vi "Assigned instruments to class.vi"(8 "error in (no error)":errorcluster, 11 "Test Framework in":refnum<class "Test Framework.lvclass">) -> (0 "error out":errorcluster, 3 "Test Framework out":refnum<class "Test Framework.lvclass">)   [LabVIEW 2020, in "Test Framework.lvclass"]
uses:
  Test Framework.lvclass
  Instruments/Instrument.lvclass
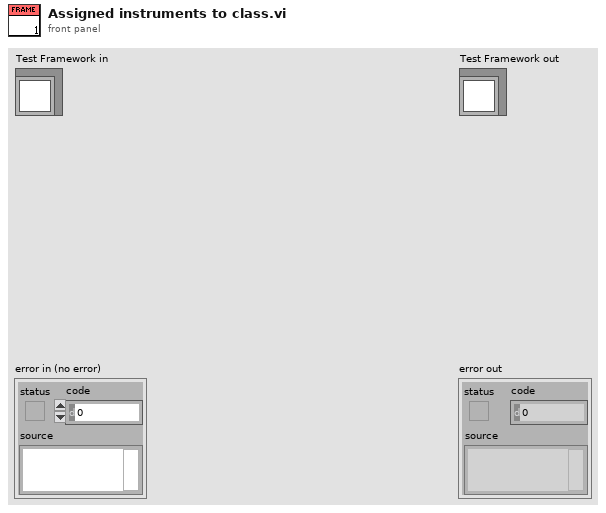
[diagram p1: front panel]
types:
  T1 = cluster{"Instrument Name":string, "Instrument.lvclass":refnum<class "Instrument.lvclass">}
  T2 = typedef "Test Framework.lvclass/Reference Selector.ctl" = enum16{"Signal Generator 1", "Signal Generator 2", "Spectrum Analyzer"}
  T3 = cluster{"Found Instruments":string[][], "Reference Selected":T2}
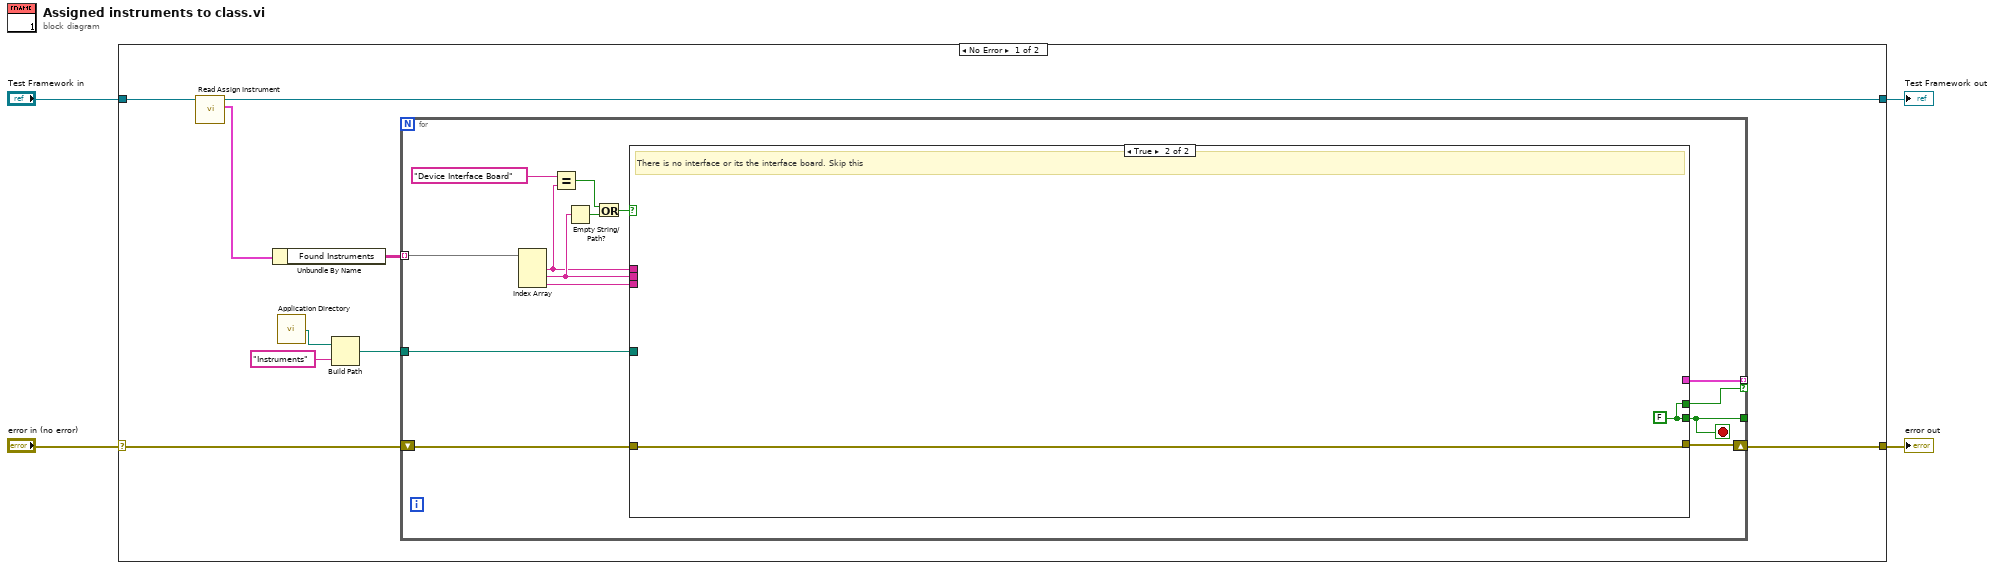
[diagram p0: block diagram]
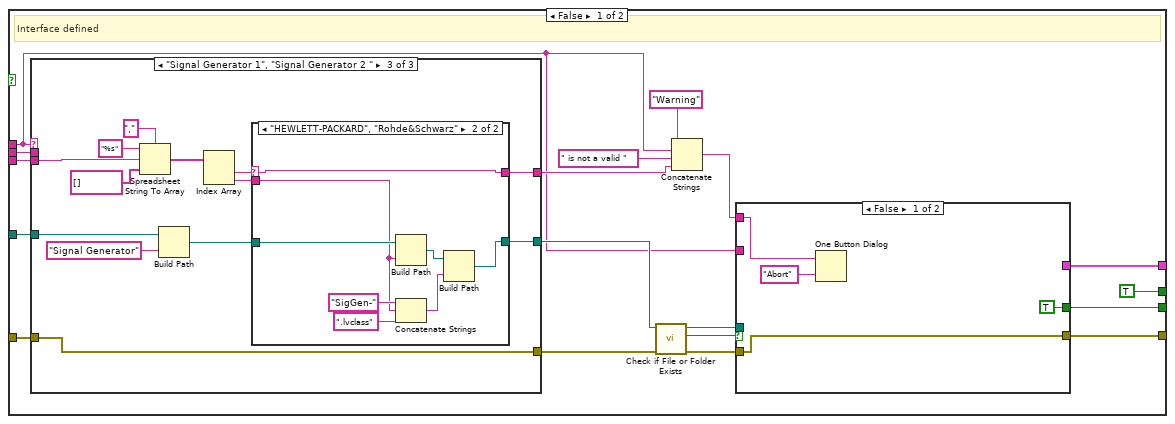
[diagram p2: hidden frame]
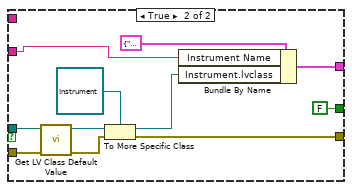
[diagram p3: hidden frame]
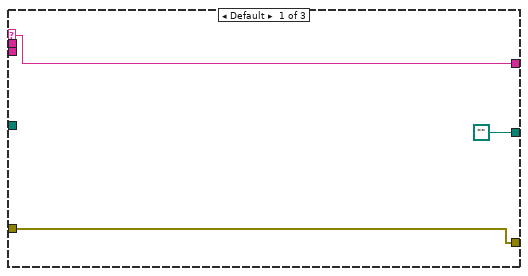
[diagram p4: hidden frame]
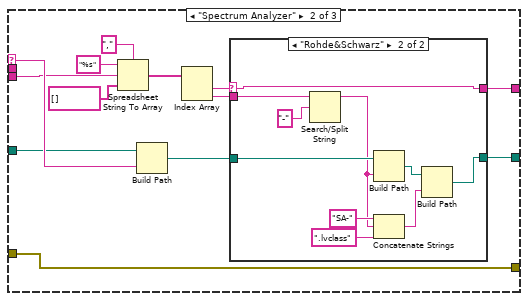
[diagram p5: hidden frame]
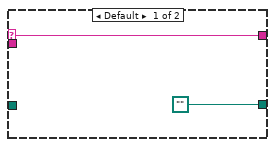
[diagram p6: hidden frame]
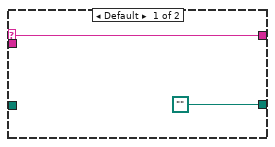
[diagram p7: hidden frame]
diagram:
  n1 = case shown="No Error" "error in (no error)" {
    selector: "error in (no error)" -> [w11 w115]
    tunnel: [w5 w115] -> w3
    tunnel: [w7 w114] -> w1
    tunnel: "Test Framework in" -> [w13 w114]
    frame No Error {
      n2 = call-dynamic "Read Assign Instrument.vi"("Test Framework in"=w13) -> ("Assign Instrument"=w6:T3, "Test Framework out"=w7:refnum<class "Test Framework.lvclass">)  [unwired: 9 in]
      n3 = Unbundle By Name(w6) -> ("Found Instruments"=w12:string[][])
      n4 = call <vilib>:"Application Directory.vi"() -> ("Application Directory"=w10:path)
      n5 = Build Path(base path=w10, name or relative path="Instruments") -> (appended path=w8:path)
      n6 = for {
        tunnel: w12 -> [w27] mode=indexing
        shift-right: [w21] -> w5
        shift-left: w11 -> [w25]
        tunnel: w8 -> [w24]
        tunnel: [w19] -> _
        tunnel: [w20] -> _ mode=indexing if=w18
        stop <- w19 stop-if-true
        n7 = Index Array(array=w27) -> (element #1=w17:string, element #2=w22:string, element #3=w26:string)  [unwired: 3 in]
        n8 = Equal?(x="Device Interface Board", y=w17) -> (x = y?=w14:bool)
        n9 = Empty String/Path?(string/path=w22) -> (empty?=w23:bool)
        n10 = Or(x=w14, y=w23) -> (x .or. y?=w15:bool)
        n11 = case shown="True" w15 {
          tunnel: w17 -> [w30 _]
          tunnel: w22 -> [w45 _]
          tunnel: w26 -> [w44 _]
          tunnel: w25 -> [w43 w113]
          tunnel: w24 -> [w42 _]
          tunnel: [w36 w113] -> w21
          tunnel: [w31 w112] -> w19
          tunnel: [w29 _] -> w20
          tunnel: [TRUE w112] -> w18
          frame False {
            # "Interface defined"
            n12 = case shown="\"Signal Generator 1\", \"Signal Generator 2 \"" w30 {
              selector: w30 -> [w63 w76 _]
              tunnel: w45 -> [_ _ _]
              tunnel: w44 -> [_ w74 w100]
              tunnel: w43 -> [w61 w65 w91]
              tunnel: w42 -> [_ w75 w101]
              tunnel: [path "" w66 w92] -> w40
              tunnel: [w61 w65 w91] -> w41
              tunnel: [w63 w64 w90] -> w33
              frame Default {
              }
              frame "Spectrum Analyzer" {
                n13 = Spreadsheet String To Array(delimiter (Tab)=",", format string="%s", spreadsheet string=w74, array type (2D Dbl)=string[] []) -> (array=w70:string[])
                n14 = Build Path(base path=w75, name or relative path=w76) -> (appended path=w67:path)
                n15 = Index Array(array=w70) -> (element #1=w69:string, element #2=w68:string)  [unwired: 2 in]
                n16 = case shown="\"Rohde&Schwarz\"" w69 {
                  selector: w69 -> [w77 w79]
                  tunnel: w68 -> [_ w88]
                  tunnel: w67 -> [_ w86]
                  tunnel: [path "" w80] -> w66
                  tunnel: [w77 w79] -> w64
                  frame Default {
                  }
                  frame "Rohde&Schwarz" {
                    n17 = Search/Split String(string=w88, search string/char (-)="-") -> (substring before match=w82:string)  [unwired: 1 in, 2 out]
                    n18 = Build Path(base path=w86, name or relative path=w82) -> (appended path=w85:path)
                    n19 = Concatenate Strings("SA-" ("string"), w82, ".lvclass" ("string")) -> (w84:string)
                    n20 = Build Path(base path=w85, name or relative path=w84) -> (appended path=w80:path)
                  }
                }
              }
              frame "Signal Generator 1", "Signal Generator 2 " {
                n21 = Spreadsheet String To Array(delimiter (Tab)=",", format string="%s", spreadsheet string=w100, array type (2D Dbl)=string[] []) -> (array=w96:string[])
                n22 = Build Path(base path=w101, name or relative path="Signal Generator") -> (appended path=w93:path)
                n23 = Index Array(array=w96) -> (element #1=w95:string, element #2=w94:string)  [unwired: 2 in]
                n24 = case shown="\"HEWLETT-PACKARD\", \"Rohde&Schwarz\"" w95 {
                  selector: w95 -> [w102 w105]
                  tunnel: w94 -> [_ w104]
                  tunnel: w93 -> [_ w111]
                  tunnel: [path "" w106] -> w92
                  tunnel: [w102 w105] -> w90
                  frame Default {
                  }
                  frame "HEWLETT-PACKARD", "Rohde&Schwarz" {
                    n25 = Build Path(base path=w111, name or relative path=w104) -> (appended path=w110:path)
                    n26 = Concatenate Strings("SigGen-" ("string"), w104, ".lvclass" ("string")) -> (w109:string)
                    n27 = Build Path(base path=w110, name or relative path=w109) -> (appended path=w106:path)
                  }
                }
              }
            }
            n28 = call <vilib>:"Check if File or Folder Exists.vi"("error in (no error)"=w41, "path"=w40) -> ("error out"=w37:errorcluster, "file or folder exists?"=w39:bool, "dup path"=w38:path)  [unwired: 7 in]
            n29 = Concatenate Strings("Warning" ("string"), w30, " is not a valid " ("string"), w33) -> (w32:string)
            n30 = case shown="False" w39 {
              tunnel: w38 -> [_ w60]
              tunnel: w37 -> [w49 w59]
              tunnel: [w49 w55] -> w36
              tunnel: w32 -> [w48 _]
              tunnel: [TRUE FALSE] -> w31
              tunnel: w30 -> [_ w52]
              tunnel: [_ w50] -> w29
              frame False {
                n31 = One Button Dialog(message=w48, button name ("OK")="Abort") -> ()  [unwired: 1 out]
              }
              frame True {
                n32 = call <vilib>:"Get LV Class Default Value.vi"("error in (no error)"=w59, "class path"=w60) -> ("error out"=w57:errorcluster, "object"=w58:refnum<class>)  [unwired: 8 in]
                n33 = To More Specific Class(target class=refnum<class "Instrument.lvclass"> refnum ("Instrument.lvclass"), reference=w58, error in=w57) -> (specific class reference=w51:refnum<class "Instrument.lvclass">, error out=w55:errorcluster)
                n34 = Bundle By Name(cluster=T1 {"Instrument Name"="", "Instrument.lvclass"=refnum} ("Instrument to Use"), "Instrument Name"=w52, "Instrument.lvclass"=w51) -> (w50:T1)
              }
            }
          }
          frame True {
            w112 = FALSE
            # "There is no interface or its the interface board. Skip this"
          }
        }
      }
    }
    frame Error {
    }
  }
  "error out" <- w3
  "Test Framework out" <- w1
